vi "GUI_pos_update.vi"(0 "reference":refnum<class "OSA.lvclass">, 2 "dataType":T3, 5 "error in (no error)":errorcluster, 7 "spectrum y unit":T2, 9 "spectrum x unit":T1) -> (14 "reference out":refnum<class "OSA.lvclass">, 16 "X":cluster{"A":dbl, "B":dbl, "B-A":dbl} {"B-A" format="%^.2e"; "B" format="%.2f"; "A" format="%.2f"}, 18 "Y":cluster{"A":dbl, "B":dbl, "B-A":dbl} caption="X" {"B-A" format="%^.2e"; "B" format="%.2f"; "A" format="%.2f"}, 19 "error out":errorcluster)   [LabVIEW 2010, in "OSA.lvclass"]
doc: "SubVI to a <B>Thorlabs_OSA_64</B> object.\n\n[GOOP 1.0]"
uses:
  OSA.lvclass
  typeDef/acq_dataType.ctl
  y_unit_GUI.ctl
  typeDef/spectrum_x_unit.ctl
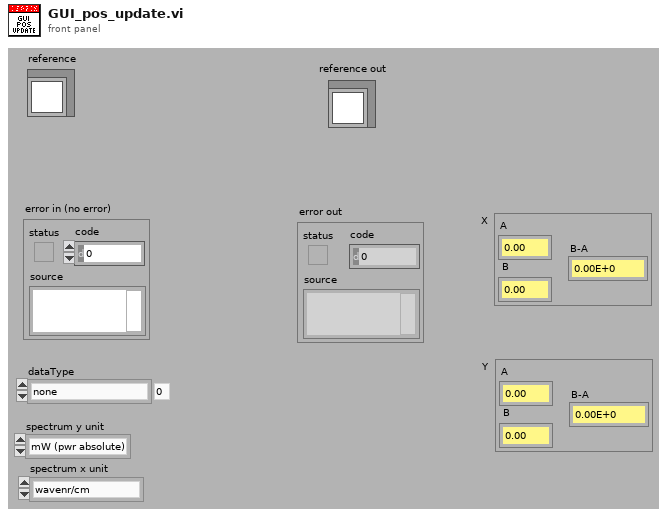
[diagram p1: front panel]
types:
  T1 = typedef "OSA.lvclass/spectrum_x_unit.ctl" = enum16{"wavenr/cm", "THz", "eV", "nm_air", "nm_vac"}
  T2 = typedef "OSA.lvclass/y_unit_GUI.ctl" = enum16{"mW (pwr absolute)", "dBm (pwr absolute)"}
  T3 = typedef "OSA.lvclass/acq_dataType.ctl" = enum16{"none", "interferogram", "spectrum"}
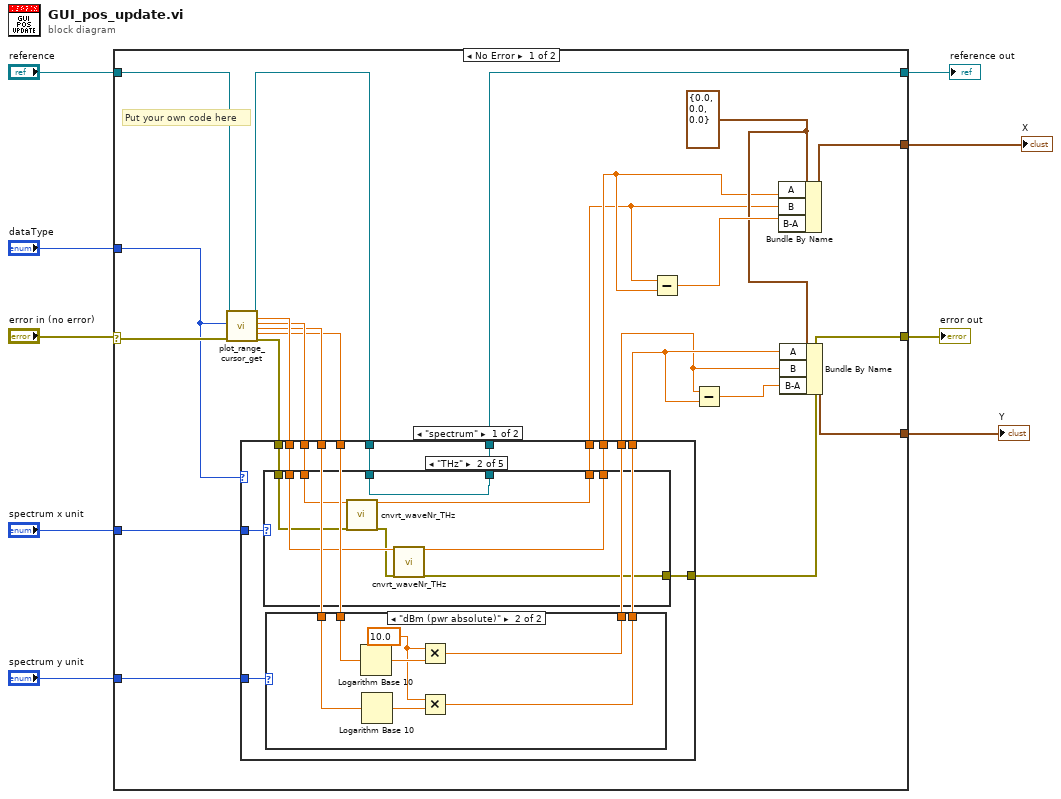
[diagram p0: block diagram]
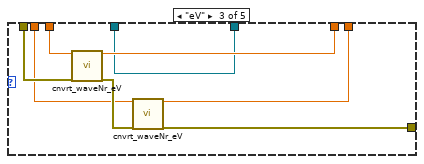
[diagram p4: hidden frame]
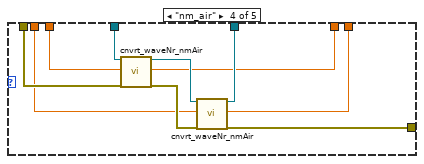
[diagram p5: hidden frame]
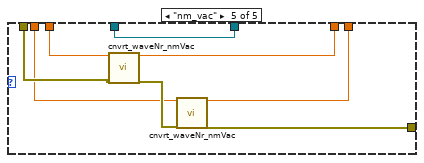
[diagram p6: hidden frame]
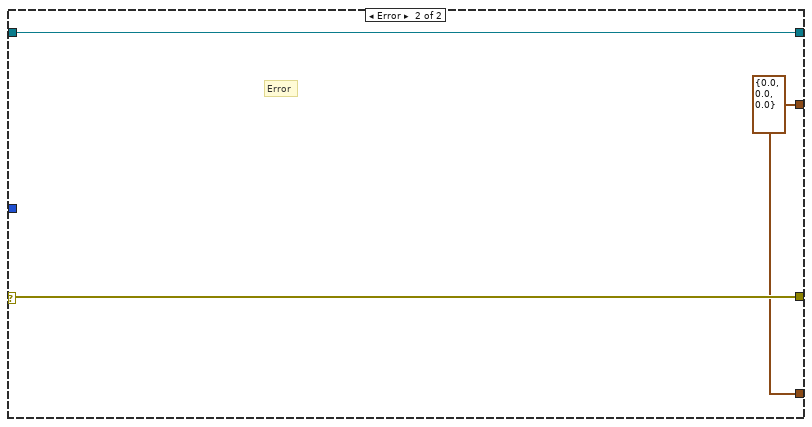
[diagram p8: hidden frame]
diagram:
  n1 = case shown="No Error" "error in (no error)" {
    selector: "error in (no error)" -> [w31 w101]
    tunnel: [w12 w101] -> w9
    tunnel: "reference" -> [w30 w100]
    tunnel: [w10 w100] -> w6
    tunnel: "dataType" -> [w24 _]
    tunnel: [w28 w99] -> w4
    tunnel: [w27 w99] -> w3
    tunnel: "spectrum y unit" -> [w22 _]
    tunnel: "spectrum x unit" -> [w23 _]
    frame No Error {
      w26 = cluster{"A":dbl, "B":dbl, "B-A":dbl} {"A"=0.0, "B"=0.0, "B-A"=0.0} ("X")
      # "Put your own code here"
      n2 = call "plot_range_cursor_get.vi"("reference"=w30, "dataType"=w24, "error in (no error)"=w31) -> ("reference out"=w11:refnum<class "OSA.lvclass">, "x min"=w21:dbl, "x max"=w19:dbl, "y min"=w16:dbl, "y max"=w14:dbl, "error out"=w13:errorcluster)  [unwired: 11 in]
      n3 = case shown="\"spectrum\"" w24 {
        tunnel: w23 -> [w45 _]
        tunnel: w21 -> [w44 w97]
        tunnel: w19 -> [w43 w96]
        tunnel: w22 -> [w42 _]
        tunnel: [w34 w97] -> w20
        tunnel: [w35 w96] -> w18
        tunnel: w16 -> [w41 w95]
        tunnel: w14 -> [w40 w94]
        tunnel: [w39 w95] -> w17
        tunnel: [w38 w94] -> w15
        tunnel: w13 -> [w36 w98]
        tunnel: [w37 w98] -> w12
        tunnel: w11 -> [w33 w93]
        tunnel: [w32 w93] -> w10
        frame "spectrum" {
          n4 = case shown="\"THz\"" w45 {
            tunnel: w44 -> [w58 w65 w69 w80 w87]
            tunnel: w43 -> [w57 w66 w74 w81 w89]
            tunnel: [w58 w63 w68 w75 w86] -> w34
            tunnel: [w57 w64 w73 w76 w88] -> w35
            tunnel: w36 -> [w56 w60 w72 w83 w92]
            tunnel: [w56 w61 w70 w84 w90] -> w37
            tunnel: w33 -> [w55 w59 w67 w79 w85]
            tunnel: [w55 w59 w67 w77 w85] -> w32
            frame "wavenr/cm", Default {
            }
            frame "THz" {
              n5 = call "cnvrt_waveNr_THz.vi"("waveNr"=w66, "error in (no error)"=w60) -> ("frequency (THz)"=w64:dbl, "error out"=w62:errorcluster)  [unwired: 16 in]
              n6 = call "cnvrt_waveNr_THz.vi"("waveNr"=w65, "error in (no error)"=w62) -> ("frequency (THz)"=w63:dbl, "error out"=w61:errorcluster)  [unwired: 16 in]
            }
            frame "eV" {
              n7 = call "cnvrt_waveNr_eV.vi"("waveNr"=w74, "error in (no error)"=w72) -> ("energy (eV)"=w73:dbl, "error out"=w71:errorcluster)  [unwired: 16 in]
              n8 = call "cnvrt_waveNr_eV.vi"("waveNr"=w69, "error in (no error)"=w71) -> ("energy (eV)"=w68:dbl, "error out"=w70:errorcluster)  [unwired: 16 in]
            }
            frame "nm_air" {
              n9 = call "cnvrt_waveNr_nmAir.vi"("reference in"=w79, "waveNr"=w81, "error in (no error)"=w83) -> ("reference out"=w78:refnum<class "OSA.lvclass">, "wavelength (nmAir)"=w76:dbl, "error out"=w82:errorcluster)  [unwired: 14 in]
              n10 = call "cnvrt_waveNr_nmAir.vi"("reference in"=w78, "waveNr"=w80, "error in (no error)"=w82) -> ("reference out"=w77:refnum<class "OSA.lvclass">, "wavelength (nmAir)"=w75:dbl, "error out"=w84:errorcluster)  [unwired: 14 in]
            }
            frame "nm_vac" {
              n11 = call "cnvrt_waveNr_nmVac.vi"("waveNr"=w89, "error in (no error)"=w92) -> ("wavelength (nmVac)"=w88:dbl, "error out"=w91:errorcluster)  [unwired: 16 in]
              n12 = call "cnvrt_waveNr_nmVac.vi"("waveNr"=w87, "error in (no error)"=w91) -> ("wavelength (nmVac)"=w86:dbl, "error out"=w90:errorcluster)  [unwired: 16 in]
            }
          }
          n13 = case shown="\"dBm (pwr absolute)\"" w42 {
            tunnel: w41 -> [w47 w54]
            tunnel: w40 -> [w46 w53]
            tunnel: [w47 w48] -> w39
            tunnel: [w46 w49] -> w38
            frame Default {
            }
            frame "dBm (pwr absolute)" {
              w50 = 10.0 ("x")
              n14 = Logarithm Base 10(1:w53) -> (0:w52:dbl)
              n15 = Logarithm Base 10(1:w54) -> (0:w51:dbl)
              n16 = Multiply(x=w50, y=w52) -> (x*y=w49:dbl)
              n17 = Multiply(x=w50, y=w51) -> (x*y=w48:dbl)
            }
          }
        }
        frame "interferogram", Default {
        }
      }
      n18 = Subtract(x=w18, y=w20) -> (x-y=w29:dbl)
      n19 = Subtract(x=w15, y=w17) -> (x-y=w25:dbl)
      n20 = Bundle By Name(cluster=w26, "A"=w20, "B"=w18, "B-A"=w29) -> (w28:cluster{"A":dbl, "B":dbl, "B-A":dbl})
      n21 = Bundle By Name(cluster=w26, "A"=w17, "B"=w15, "B-A"=w25) -> (w27:cluster{"A":dbl, "B":dbl, "B-A":dbl})
    }
    frame Error {
      w99 = cluster{"A":dbl, "B":dbl, "A-B":dbl} {"A"=0.0, "B"=0.0, "A-B"=0.0} ("X")
      # "Error"
    }
  }
  "error out" <- w9
  "reference out" <- w6
  "X" <- w4
  "Y" <- w3
